vi "KG id.vi"(8 "Fehler (Eingang, kein Fehler)":errorcluster, 11 "VISA-Ressourcenname":refnum<visa-resource-name>) -> (0 "Fehler (Ausgang)":errorcluster, 1 "Kommando gesendet":string, 2 "Id":string, 3 "VISA-Ressourcenname (Ausgang)":refnum<visa-resource-name>)   [LabVIEW 2020, in "Linearisierung v2.lvlib" / "Gasteiler.lvlib" / "HovaCAL_Interface.lvlib" / "KGN.lvlib" / "get.lvlib"]
uses:
  get.lvlib
  KGN.lvlib
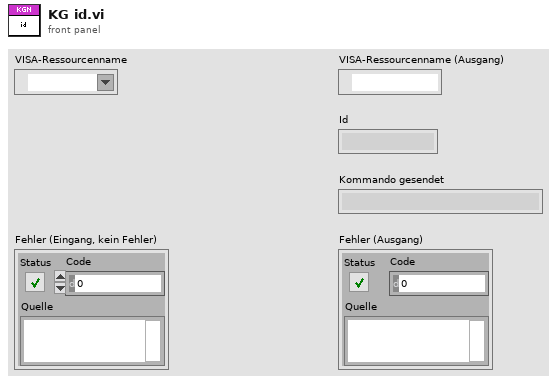
[diagram p1: front panel]
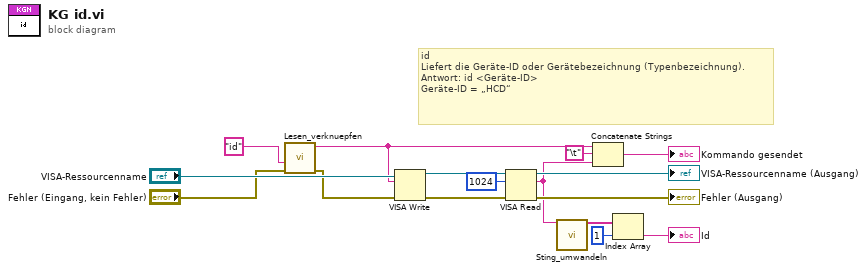
[diagram p0: block diagram]
diagram:
  # "id\nLiefert die Geräte-ID oder Gerätebezeichnung (Typenbezeichnung).\nAntwort: id <Geräte-ID>\nGeräte-ID = „HCD“"
  n1 = call "Lesen_verknuepfen.vi"("error in (no error)"="Fehler (Eingang, kein Fehler)", "Order"="id" ("Schreibpuffer")) -> ("error out"=w9:errorcluster, "Verknüpfter String"=w8:string)  [unwired: 8 in]
  n2 = VISA Write(VISA resource name="VISA-Ressourcenname", write buffer=w8, error in (no error)=w9) -> (VISA resource name out=w16:refnum<visa-resource-name>, error out=w15:errorcluster)  [unwired: 1 out]
  n3 = VISA Read(VISA resource name=w16, byte count=u32 1024 ("Byte-Anzahl"), error in (no error)=w15) -> (VISA resource name out=→"VISA-Ressourcenname (Ausgang)":refnum<visa-resource-name>, read buffer=w2:string, error out=→"Fehler (Ausgang)":errorcluster)  [unwired: 1 out]
  n4 = call "Sting_umwandeln.vi"("Lesepuffer"=w2) -> ("string array"=w6:string[])  [unwired: 8 in, 6 out]
  n5 = Concatenate Strings(w8, "\t", w2) -> (→"Kommando gesendet":string)
  n6 = Index Array(array=w6, index=1 ("Index")) -> (element=→"Id":string)
